vi "Test Inset.vi"() -> ()   [LabVIEW 2019]
uses:
  Parse/ParseXML/ParseSVG.lvclass
  Parse/ParseVectorFile/ParseVectorFile.lvclass
  Inset.lvclass
  Parse/ParseXML/ParseSVG.lvclass/ParseSVG.ctl
  Parse/Image/SVGImage.lvclass
  C:/Users/Albro/Documents/GitHub/AFM-Lithography/lvsrc/Classes/Parse/SVG Object/SVG Object.lvclass
  BigMAQ/BigMAQ.lvclass
panel:
  in  "Background Path":path=path "C:/Users/Albro/Documents/GitHub/AFM-Lithography/test files/SA01234A0000.ibw"
  in  "Collapse":bool
  out "Render":T1(plugin-control)
  in  "Inkscape Path":path
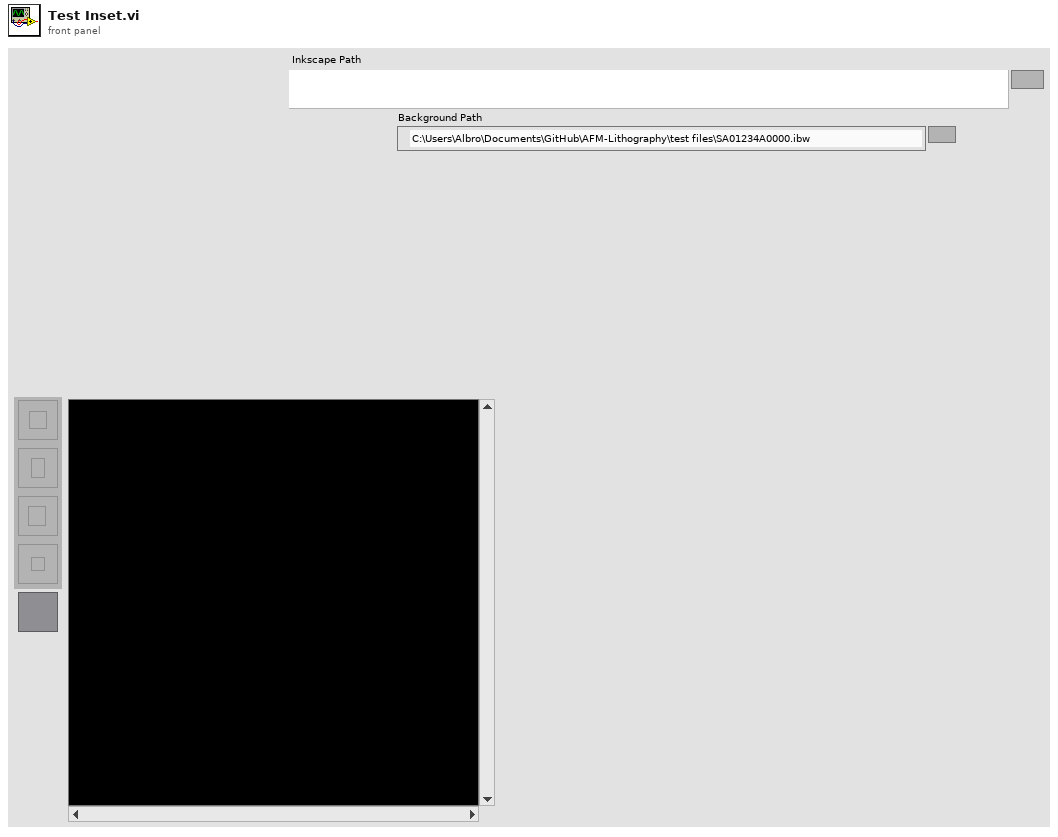
[diagram p1: front panel]
types:
  T1 = typedef "IMAQ Image.ctl" = refnum<image>
  T2 = cluster{"Background.Range":cluster{sgl, sgl}, "Background.Page":i32}
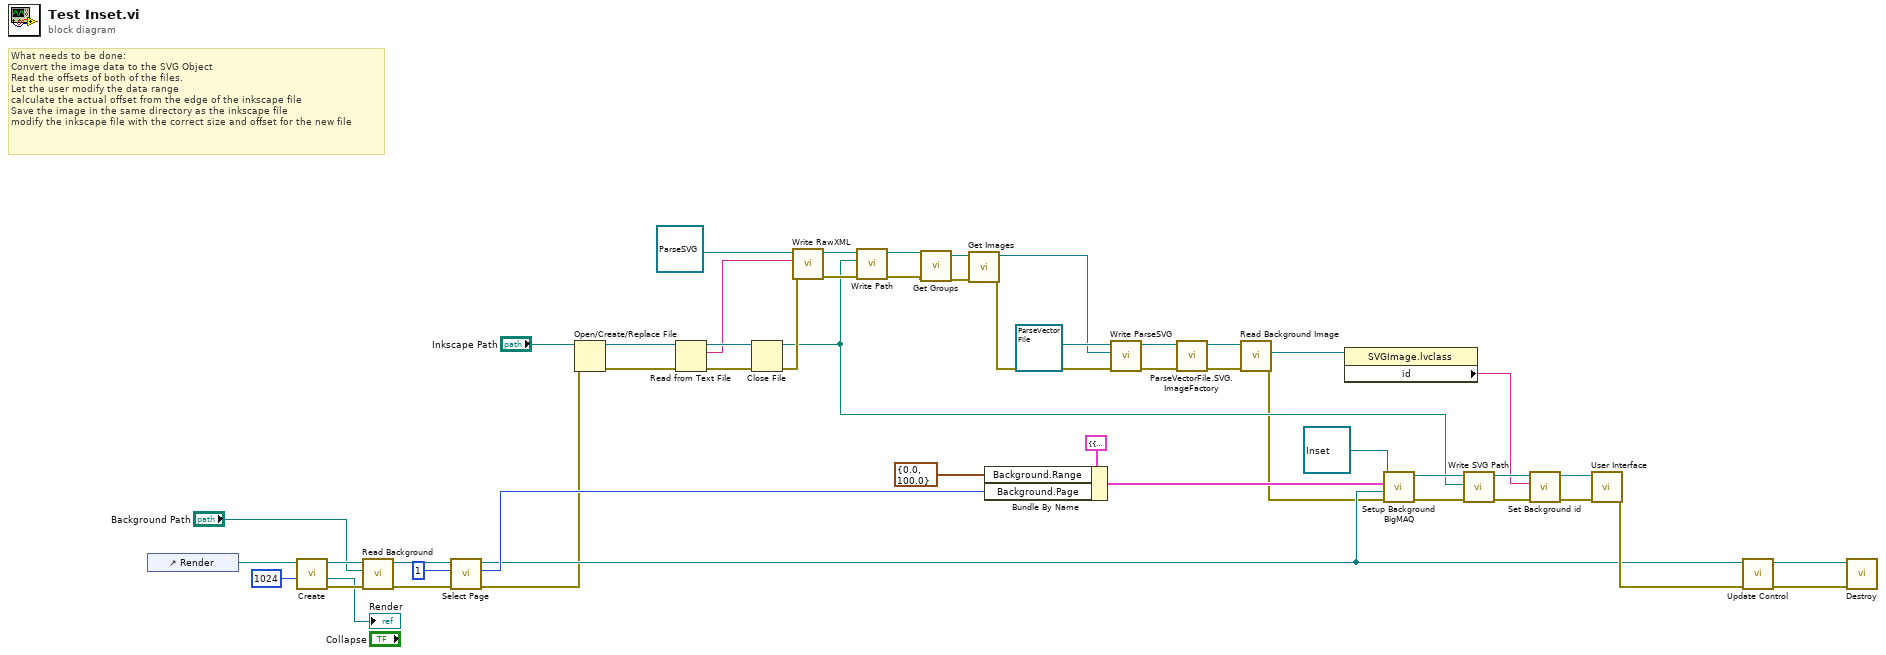
[diagram p0: block diagram]
diagram:
  # "What needs to be done:\nConvert the image data to the SVG Object\nRead the offsets of both of the files.\nLet the user modify the data range\ncalculate the actual offset from the edge of the inkscape file\nSave the image in the same directory as the inkscape file\nmodify the inkscape file with the correct size and offset for the new file"
  n1 = control-ref of="Render"() -> (w36:refnum<vi>)
  n2 = call "Create.vi"("Resolution"=1024, "Reference"=w36) -> ("error out"=w37:errorcluster, "To Control"=→"Render":T1, "BigMAQ out"=w38:refnum<class "BigMAQ.lvclass">)  [unwired: 7 in]
  n3 = call "Read Background.vi"("error in (no error)"=w37, "Path"="Background Path", "BigMAQ in"=w38) -> ("error out"=w33:errorcluster, "BigMAQ out"=w32:refnum<class "BigMAQ.lvclass">)  [unwired: 6 in, 1 out]
  n4 = call "Select Page.vi"("error in (no error)"=w33, "Page"=1, "BigMAQ in"=w32) -> ("error out"=w3:errorcluster, "Corrected Page"=w6:u32, "BigMAQ out"=w5:refnum<class "BigMAQ.lvclass">)  [unwired: 6 in]
  n5 = Open/Create/Replace File(file path (use dialog)="Inkscape Path", error in=w3) -> (refnum out=w45:refnum<file>, error out=w11:errorcluster)  [unwired: 4 in, 1 out]
  n6 = Read from Text File(file (use dialog)=w45, error in=w11) -> (refnum out=w44:refnum<file>, text=w39:string, error out=w43:errorcluster)  [unwired: 2 in, 1 out]
  n7 = Close File(refnum=w44, error in=w43) -> (path=w2:path, error out=w13:errorcluster)
  n8 = call "Write RawXML.vi"("error in (no error)"=w13, "RawXML"=w39, "ParseSVG.lvclass"=refnum<class "ParseSVG.lvclass"> refnum ("ParseSVG in")) -> ("error out"=w17:errorcluster, "ParseSVG.lvclass 2"=w16:refnum<class "ParseSVG.lvclass">)  [unwired: 7 in]
  n9 = call-dynamic "Write Path.vi"("error in (no error)"=w17, "Path"=w2, "ParseSVG in"=w16) -> ("error out"=w18:errorcluster, "ParseSVG out"=w15:refnum<class "ParseSVG.lvclass">)  [unwired: 7 in]
  n10 = call "Get Groups.vi"("error in (no error)"=w18, "ParseSVG in"=w15) -> ("error out"=w49:errorcluster, "ParseSVG out"=w50:refnum<class "ParseSVG.lvclass">)  [unwired: 8 in]
  n11 = call "Get Images.vi"("error in (no error)"=w49, "ParseSVG in"=w50) -> ("error out"=w12:errorcluster, "ParseSVG out"=w40:refnum<class "ParseSVG.lvclass">)  [unwired: 8 in]
  n12 = Bundle By Name(cluster=T2 {"Background.Range"={0.0, 100.0}, "Background.Page"=0} ("Display Settings"), "Background.Range"=cluster{sgl, sgl} {0.0, 100.0}, "Background.Page"=w6) -> (w27:T2)
  n13 = call-dynamic "Write ParseSVG.vi"("error in (no error)"=w12, "ParseSVG.lvclass"=w40, "ParseVectorFile in"=refnum<class "ParseVectorFile.lvclass"> refnum ("ParseVectorFile.lvclass")) -> ("error out"=w46:errorcluster, "ParseVectorFile out"=w47:refnum<class "ParseVectorFile.lvclass">)  [unwired: 7 in]
  n14 = call "ParseVectorFile.SVG.ImageFactory.vi"("error in (no error)"=w46, "ParseVectorFile in"=w47) -> ("error out"=w41:errorcluster, "ParseVectorFile out"=w42:refnum<class "ParseVectorFile.lvclass">)  [unwired: 8 in]
  n15 = call-dynamic "Read Background Image.vi"("error in (no error)"=w41, "ParseVectorFile in"=w42) -> ("error out"=w1:errorcluster, "SVGImage.lvclass"=w22:refnum<class "SVGImage.lvclass">)  [unwired: 7 in, 1 out]
  n16 = property class="SVGImage.lvclass"(reference=w22) -> ("id"=w4:string)  [unwired: 1 in, 2 out]
  n17 = call "Setup Background BigMAQ.vi"("error in"=w1, "BigMAQ"=w5, "Display Settings"=w27, "Inset in"=refnum<class "Inset.lvclass"> refnum) -> ("error out"=w9:errorcluster, "Inset out"=w25:refnum<class "Inset.lvclass">)  [unwired: 6 in]
  n18 = call "Write SVG Path.vi"("error in"=w9, "Path"=w2, "Inset in"=w25) -> ("error out"=w8:errorcluster, "Inset out"=w24:refnum<class "Inset.lvclass">)  [unwired: 7 in]
  n19 = call "Set Background id.vi"("error in"=w8, "id"=w4, "Inset in"=w24) -> ("error out"=w7:errorcluster, "Inset out"=w23:refnum<class "Inset.lvclass">)  [unwired: 7 in]
  n20 = call "User Interface.vi"("error in"=w7, "Inset In"=w23) -> ("error out"=w31:errorcluster)  [unwired: 8 in, 1 out]
  n21 = call "Update Control.vi"("error in"=w31, "BigMAQ in"=w5) -> ("error out"=w21:errorcluster, "BigMAQ out"=w20:refnum<class "BigMAQ.lvclass">)  [unwired: 8 in]
  n22 = call "Destroy.vi"("error in"=w21, "BigMAQ in"=w20) -> ()  [unwired: 8 in, 2 out]
